vi "_StartLCRun.vi"() -> (1 "No LC":bool, 2 "error out":errorcluster)   [LabVIEW 2012]
uses:
  Type/_XML Type.ctl
  Type/_Log Command.ctl
  Type/_LC Command.ctl
  Configuration/_Global Configuration.vi
  LCDriver/_Global LC Driver.vi
  _Server Global.vi
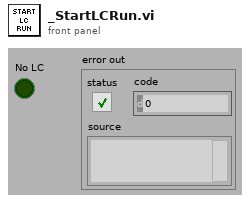
[diagram p1: front panel]
types:
  T1 = typedef "_XML Type.ctl" = enum16{"Configuration", "ConTable", "Method", "Experiment", "Mass Range", "Table", "LensTable", "ParamTable", "TuneParam", "MetParam", "MassRange", "LCMethod", "LCMethodFile", "RackType", "Vial", "PlatePos", "InjVol"}
  T2 = typedef "_Log Command.ctl" = enum16{"No Command", "Open", "Read", "Write", "Close", "Check Size"}
  T3 = typedef "_LC Command.ctl" = enum16{"No Command", "Initialize", "Get Configuration", "Get Status", "Get LC Method Contents", "Oven OnOff", "Pump OnOFF", "Rinse Autosampler", "Run Sample", "Set EnvParameters", "Set Method", "Start Equilibration", "Stop Run", "Get LastError", "Clear Error", "Close"}
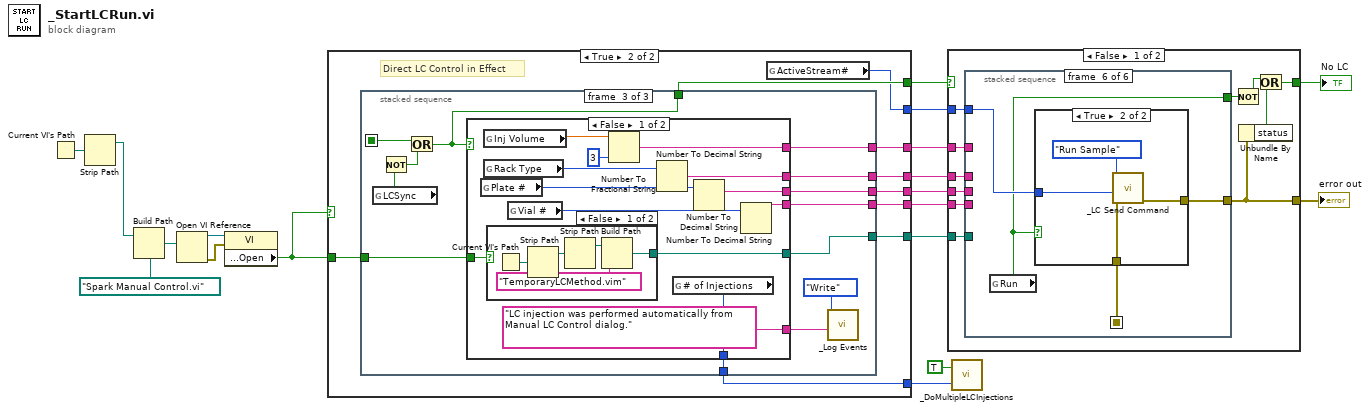
[diagram p0: block diagram]
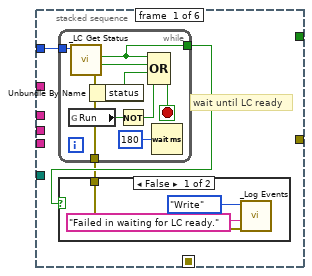
[diagram p2: hidden frame]
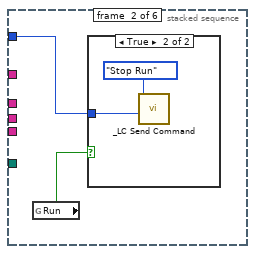
[diagram p4: hidden frame]
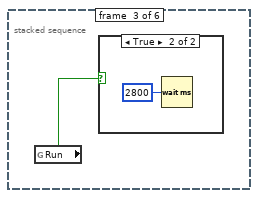
[diagram p6: hidden frame]
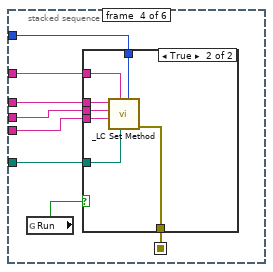
[diagram p8: hidden frame]
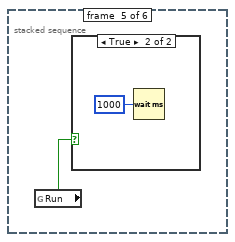
[diagram p10: hidden frame]
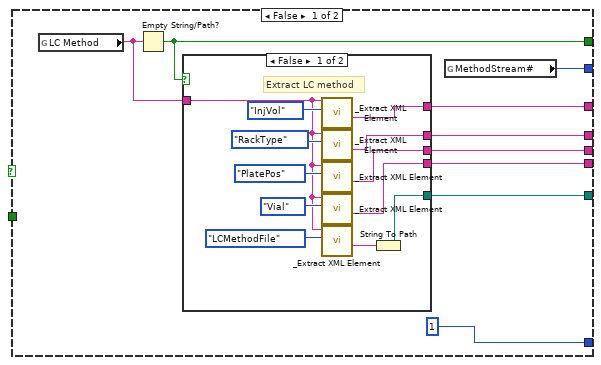
[diagram p14: hidden frame]
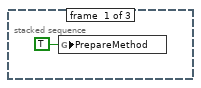
[diagram p16: hidden frame]
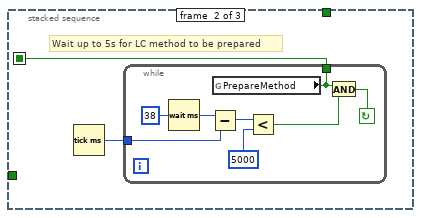
[diagram p17: hidden frame]
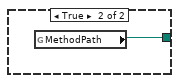
[diagram p18: hidden frame]
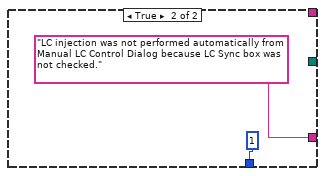
[diagram p19: hidden frame]
diagram:
  n1 = Current VI's Path() -> (path=w18:path)
  n2 = Strip Path(path=w18) -> (stripped path=w3:path)  [unwired: 1 out]
  n3 = Build Path(base path=w3, name or relative path=path "Spark Manual Control.vi") -> (appended path=w4:path)
  n4 = Open VI Reference(vi path=w4) -> (vi reference=w5:refnum<vi>, error out=w6:errorcluster)  [unwired: 1 in, 4 out]
  n5 = property class="VI"(reference=w5, error in=w6) -> ("Front Panel.Open"=w1:bool)  [unwired: 2 out]
  n6 = case shown="True" w1 {
    tunnel: [w22 w48] -> w13
    tunnel: [w24 w47] -> w15
    tunnel: [w25 w46] -> w16
    tunnel: [w23 w45] -> w14
    tunnel: [w27 w44] -> w17
    tunnel: [w21 w42] -> w12
    tunnel: [u16 1 ("# of Injections") w43] -> w11
    tunnel: w1 -> [_ w41]
    tunnel: [w19 w40] -> w2
    frame False {
      n7 = global read "_Global Configuration.vi" "LC Method"() -> (w26:string)
      n8 = Empty String/Path?(string/path=w26) -> (empty?=w27:bool)
      n9 = case shown="False" w27 {
        tunnel: w26 -> [w33 _]
        tunnel: [w32 _] -> w25
        tunnel: [w31 _] -> w24
        tunnel: [w30 _] -> w23
        tunnel: [w29 _] -> w22
        tunnel: [w28 _] -> w21
        frame False {
          # "Extract LC method"
          n10 = call "_Extract XML Element.vi"("XML Type"=_XML_Type."InjVol", "XML String"=w33) -> ("Element"=w32:string)  [unwired: 1 in, 4 out]
          n11 = call "_Extract XML Element.vi"("XML Type"=_XML_Type."RackType", "XML String"=w33) -> ("Element"=w31:string)  [unwired: 1 in, 4 out]
          n12 = call "_Extract XML Element.vi"("XML Type"=_XML_Type."PlatePos", "XML String"=w33) -> ("Element"=w28:string)  [unwired: 1 in, 4 out]
          n13 = call "_Extract XML Element.vi"("XML Type"=_XML_Type."Vial", "XML String"=w33) -> ("Element"=w30:string)  [unwired: 1 in, 4 out]
          n14 = call "_Extract XML Element.vi"("XML Type"=_XML_Type."LCMethodFile", "XML String"=w33) -> ("Element"=w34:string)  [unwired: 1 in, 4 out]
          n15 = String To Path(string=w34) -> (path=w29:path)
        }
        frame True {
        }
      }
      n16 = global read "_Global LC Driver.vi" "MethodStream#"() -> (w19:u8)
    }
    frame True {
      # "Direct LC Control in Effect"
      n17 = stacked-sequence {
        seq-local: [_ w50 _] -> [_ _ w66]
        tunnel: [_ _ w72] -> w48
        tunnel: [_ _ w71] -> w46
        tunnel: [_ _ w70] -> w47
        tunnel: [_ _ w69] -> w45
        tunnel: [_ _ w64] -> w44
        tunnel: [_ _ w68] -> w43
        tunnel: [_ _ w61] -> w42
        tunnel: w41 -> [_ _ w60]
        frame #0 {
          n18 = global write "_Server Global.vi" "PrepareMethod"(TRUE ("PrepareMethod")) -> ()
        }
        frame #1 {
          # "Wait up to 5s for LC method to be prepared"
          n19 = Tick Count (ms)() -> (millisecond timer value=w51:u32)
          n20 = while {
            tunnel: w51 -> [w56]
            tunnel: [w52] -> w50
            stop <- w59 continue-if-true
            n21 = Wait (ms)(milliseconds to wait=u32 38) -> (millisecond timer value=w57:u32)
            n22 = Subtract(x=w57, y=w56) -> (x-y=w55:u32)
            n23 = global read "_Server Global.vi" "PrepareMethod"() -> (w52:bool)
            n24 = Less?(x=w55, y=u32 5000) -> (x < y?=w53:bool)
            n25 = And(x=w52, y=w53) -> (x .and. y?=w59:bool)
          }
        }
        frame #2 {
          n26 = global read "_Server Global.vi" "LCSync"() -> (w67:bool)
          n27 = Not(x=w67) -> (.not. x?=w65:bool)
          n28 = Or(x=w66, y=w65) -> (x .or. y?=w64:bool)
          n29 = case shown="False" w64 {
            tunnel: [w85 _] -> w72
            tunnel: [w80 _] -> w71
            tunnel: [w79 _] -> w70
            tunnel: [w78 _] -> w69
            tunnel: [w77 u16 1 ("# of Injections")] -> w68
            tunnel: ["LC injection was performed automatically from Manual LC Control dialog." "LC injection was not performed automatically from Manual LC Control Dialog because LC Sync box was not checked."] -> w62
            tunnel: [w74 _] -> w61
            tunnel: w60 -> [w73 _]
            frame False {
              n30 = global read "_Server Global.vi" "Plate #"() -> (w75:u16)
              n31 = global read "_Server Global.vi" "Inj Volume"() -> (w84:dbl)
              n32 = global read "_Server Global.vi" "Rack Type"() -> (w82:u16)
              n33 = case shown="False" w73 {
                tunnel: [w86 w91] -> w85
                frame False {
                  n34 = Current VI's Path() -> (path=w87:path)
                  n35 = Strip Path(path=w87) -> (stripped path=w88:path)  [unwired: 1 out]
                  n36 = Strip Path(path=w88) -> (stripped path=w89:path)  [unwired: 1 out]
                  n37 = Build Path(base path=w89, name or relative path="TemporaryLCMethod.vim" ("extension (isd)")) -> (appended path=w86:path)
                }
                frame True {
                  n38 = global read "_Server Global.vi" "MethodPath"() -> (w91:path)
                }
              }
              n39 = global read "_Server Global.vi" "Vial #"() -> (w81:u16)
              n40 = Number To Fractional String(number=w84, precision (6)=i16 3) -> (F-format string=w80:string)  [unwired: 2 in]
              n41 = Number To Decimal String(number=w82) -> (decimal integer string=w79:string)  [unwired: 1 in]
              n42 = global read "_Server Global.vi" "# of Injections"() -> (w77:u16)
              n43 = Number To Decimal String(number=w75) -> (decimal integer string=w74:string)  [unwired: 1 in]
              n44 = Number To Decimal String(number=w81) -> (decimal integer string=w78:string)  [unwired: 1 in]
            }
            frame True {
            }
          }
          n45 = call "_Log Events.vi"("Event"=w62, "Log Command"=_Log_Command."Write") -> ()  [unwired: 5 in, 2 out]
        }
      }
      n46 = global read "_Global LC Driver.vi" "ActiveStream#"() -> (w40:u8)
    }
  }
  n47 = case shown="False" w17 {
    selector: w17 -> [_ w152]
    tunnel: w16 -> [w104 _]
    tunnel: w15 -> [w103 _]
    tunnel: w14 -> [w102 _]
    tunnel: w13 -> [w101 _]
    tunnel: w12 -> [w100 _]
    tunnel: [w96 w152] -> w9
    tunnel: [w99 _] -> w8
    tunnel: w2 -> [w98 _]
    frame False {
      n48 = stacked-sequence {
        seq-local: [_ _ _ w128 _ _] -> [_ _ _ _ _ w146]
        tunnel: w104 -> [_ _ _ w133 _ _]
        tunnel: w103 -> [_ _ _ w132 _ _]
        tunnel: w102 -> [_ _ _ w131 _ _]
        tunnel: w101 -> [_ _ _ w130 _ _]
        tunnel: w100 -> [_ _ _ w129 _ _]
        tunnel: [_ _ _ _ _ w145] -> w99
        tunnel: w98 -> [w107 w121 _ w127 _ w144]
        tunnel: [_ _ _ _ _ w143] -> w97
        frame #0 {
          # "wait until LC ready"
          n49 = while {
            tunnel: w107 -> [w113]
            tunnel: [w112] -> w106
            tunnel: [w111] -> w105
            stop <- w117 stop-if-true
            n50 = global read "_Global Configuration.vi" "Run"() -> (w116:bool)
            n51 = call "_LC Get Status.vi"("Stream#"=w113) -> ("error out"=w111:errorcluster, "Error"=w118:bool, "Ready"=w112:bool)  [unwired: 3 in, 2 out]
            n52 = Unbundle By Name(w111) -> ("status"=w115:bool)
            n53 = Not(x=w116) -> (.not. x?=w114:bool)
            n54 = Compound Arithmetic op=OR(w112, w118, w115, w114) -> (w117:bool)
            n55 = Wait (ms)(milliseconds to wait=u32 180) -> ()  [unwired: 1 out]
          }
          n56 = case shown="False" w106 {
            tunnel: w105 -> [w109 _]
            frame False {
              n57 = call "_Log Events.vi"("error in (no error)"=w109, "Event"="Failed in waiting for LC ready.", "Log Command"=_Log_Command."Write") -> ()  [unwired: 1 in, 5 out]
            }
            frame True {
            }
          }
        }
        frame #1 {
          n58 = global read "_Global Configuration.vi" "Run"() -> (w120:bool)
          n59 = case shown="True" w120 {
            tunnel: w121 -> [_ w122]
            frame False {
            }
            frame True {
              n60 = call "_LC Send Command.vi"("Stream#"=w122, "Command"=_LC_Command."Stop Run") -> ()  [unwired: 8 in, 2 out]
            }
          }
        }
        frame #2 {
          n61 = global read "_Global Configuration.vi" "Run"() -> (w124:bool)
          n62 = case shown="True" w124 {
            frame False {
            }
            frame True {
              n63 = Wait (ms)(milliseconds to wait=u32 2800) -> ()  [unwired: 1 out]
            }
          }
        }
        frame #3 {
          n64 = global read "_Global Configuration.vi" "Run"() -> (w126:bool)
          n65 = case shown="True" w126 {
            tunnel: w133 -> [_ w140]
            tunnel: w132 -> [_ w139]
            tunnel: w131 -> [_ w138]
            tunnel: w130 -> [_ w137]
            tunnel: w129 -> [_ w136]
            tunnel: [_ w135] -> w128
            tunnel: w127 -> [_ w134]
            frame False {
            }
            frame True {
              n66 = call "_LC Set Method.vi"("Stream#"=w134, "Path"=w137, "Injection Volume"=w140, "Vial Number"=w138, "Plate Number"=w136, "Rack Type"=w139) -> ("error out"=w135:errorcluster)  [unwired: 1 in, 4 out]
            }
          }
        }
        frame #4 {
          n67 = global read "_Global Configuration.vi" "Run"() -> (w141:bool)
          n68 = case shown="True" w141 {
            frame False {
            }
            frame True {
              n69 = Wait (ms)(milliseconds to wait=u32 1000) -> ()  [unwired: 1 out]
            }
          }
        }
        frame #5 {
          n70 = global read "_Global Configuration.vi" "Run"() -> (w143:bool)
          n71 = case shown="True" w143 {
            tunnel: w146 -> [w147 w150]
            tunnel: [w147 w149] -> w145
            tunnel: w144 -> [_ w148]
            frame False {
            }
            frame True {
              n72 = call "_LC Send Command.vi"("error in"=w150, "Stream#"=w148, "Command"=_LC_Command."Run Sample") -> ("error out"=w149:errorcluster)  [unwired: 7 in, 1 out]
            }
          }
        }
      }
      n73 = Not(x=w97) -> (.not. x?=w95:bool)
      n74 = Unbundle By Name(w99) -> ("status"=w94:bool)
      n75 = Or(x=w95, y=w94) -> (x .or. y?=w96:bool)
    }
    frame True {
    }
  }
  "No LC" <- w9
  "error out" <- w8
  n76 = call "_DoMultipleLCInjections.vi"("# of Injections"=w11, "FirstCall (F)"=TRUE) -> ()  [unwired: 2 in]
